vi "Read subindex (bool).vi"(8 "error in":errorcluster, 11 "Modbus Module Channel in":refnum<class "Modbus Module Channel.lvclass">) -> (0 "error out":errorcluster, 2 "subindex (bool)":i32, 3 "Modbus Module Channel out":refnum<class "Modbus Module Channel.lvclass">)   [LabVIEW 2015, in "Modbus Module Channel.lvclass"]
uses:
  Modbus Module Channel.lvclass
  Modbus Module Channel.lvclass/Modbus Module Channel.ctl
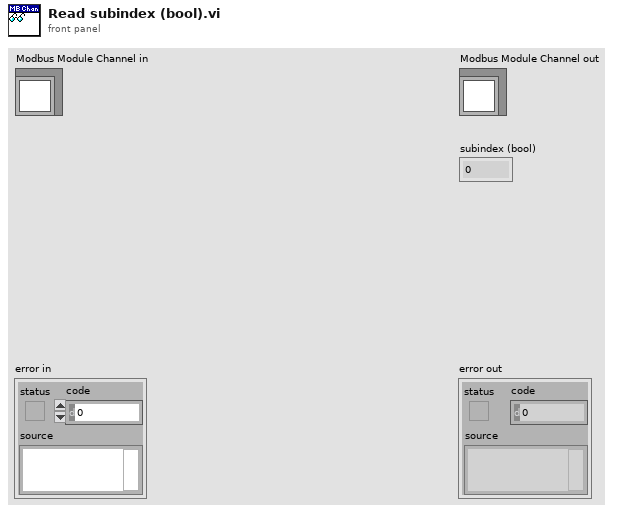
[diagram p1: front panel]
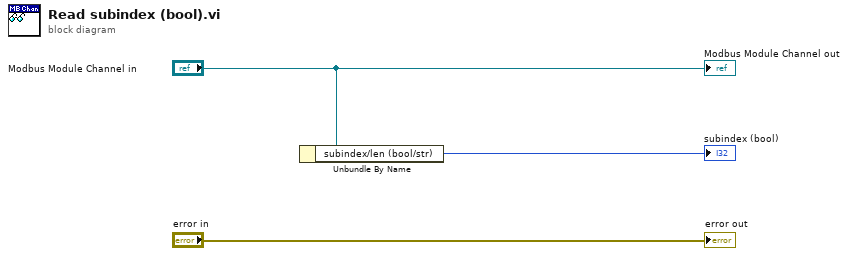
[diagram p0: block diagram]
diagram:
  n1 = Unbundle By Name("Modbus Module Channel in") -> ("subindex/len (bool/str)"=→"subindex (bool)":i32)
  "error out" <- "error in"
  "Modbus Module Channel out" <- "Modbus Module Channel in"
